vi "WASH communication handler.vi"(7 "task":T2, 8 "error in (no error)":errorcluster, 11 "parameters":variant) -> (0 "error out":errorcluster, 1 "timed out?":bool, 2 "UI data":variant, 3 "UI command":T1)   [LabVIEW 2013]
doc: "Handles communication between controller and console/consoles. It separates controller from console. In subsequent phases of the project only this VI has to be modified to establish communication between controller and the console.\n\n[Covers: SI1]"
uses:
  type defs/WASH communication module tasks.ctl
  type defs/WASH UI to CTRL commands.ctl
  type defs/Wash CTRL to UI message.ctl
  type defs/WASH CTRL to UI commands.ctl
  type defs/WASH UI to CTRL message.ctl
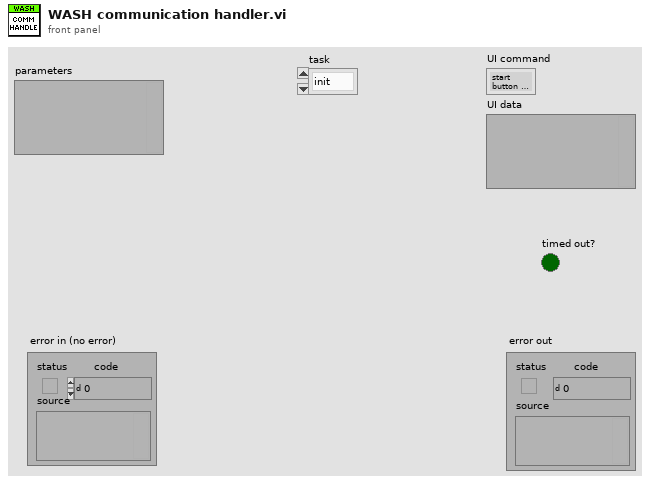
[diagram p1: front panel]
types:
  T1 = typedef "WASH UI to CTRL commands.ctl" = enum16{"start button pushed", "vehicle position changed"}
  T2 = typedef "WASH communication module tasks.ctl" = enum16{"init", "enable controls", "update wash indicators", "update wash entry", "update vehicle out of pos", "update timing", "set step buttons values", "set start button value", "set vehicle position entry", "wait for input", "close"}
  T3 = typedef "Wash CTRL to UI message.ctl" = cluster{"command":T4, "data":variant}
  T4 = typedef "WASH CTRL to UI commands.ctl" = enum16{"enable controls", "set start button value", "update vehicle out of pos", "update wash indicators", "update timing", "set vehicle position entry", "abort"}
  T5 = typedef "WASH UI to CTRL message.ctl" = cluster{"command":T1, "data":variant}
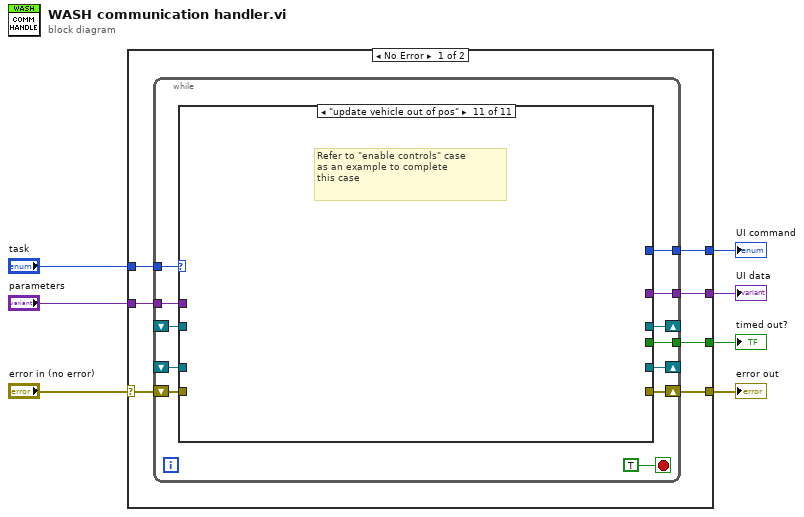
[diagram p0: block diagram]
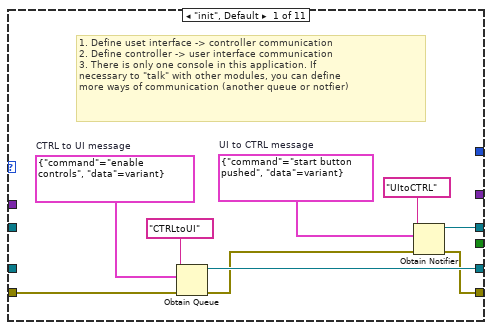
[diagram p2: hidden frame]
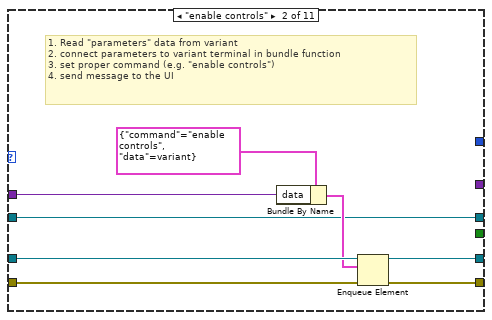
[diagram p3: hidden frame]
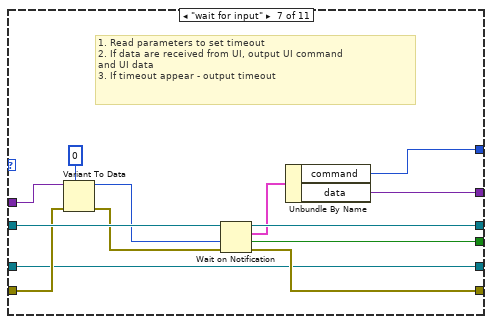
[diagram p8: hidden frame]
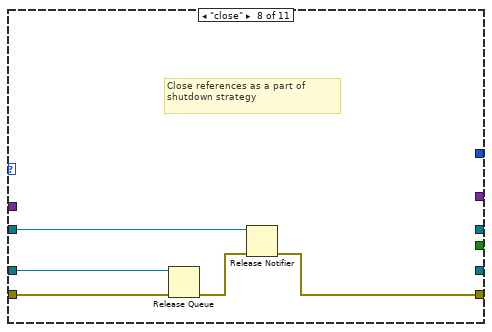
[diagram p9: hidden frame]
diagram:
  n1 = case shown="No Error" "error in (no error)" {
    selector: "error in (no error)" -> [w13 w62]
    tunnel: [w12 w62] -> w6
    tunnel: "task" -> [w14 _]
    tunnel: "parameters" -> [w11 _]
    tunnel: [w10 _] -> w3
    tunnel: [w9 _] -> w2
    tunnel: [w8 _] -> w1
    frame No Error {
      n2 = while {
        tunnel: w14 -> [w25]
        shift-right: [w24] -> _
        shift-left: _ -> [w18]
        shift-right: [w23] -> _
        shift-left: _ -> [w20]
        shift-right: [w21] -> w12
        shift-left: w13 -> [w22]
        tunnel: w11 -> [w19]
        tunnel: [w17] -> w10
        tunnel: [w16] -> w9
        tunnel: [w15] -> w8
        stop <- TRUE stop-if-true
        n3 = case shown="\"update vehicle out of pos\"" w25 {
          tunnel: [w35 w36 _ _ _ _ w55 _ _ _ _] -> w24
          tunnel: [w34 w42 _ _ _ _ w44 _ _ _ _] -> w23
          tunnel: w22 -> [w32 w41 _ _ _ _ w52 w59 _ _ _]
          tunnel: [w31 w40 _ _ _ _ w54 w57 _ _ _] -> w21
          tunnel: w20 -> [_ w43 _ _ _ _ w44 w60 _ _ _]
          tunnel: w19 -> [_ w38 _ _ _ _ w53 _ _ _ _]
          tunnel: w18 -> [_ w36 _ _ _ _ w56 w61 _ _ _]
          tunnel: [_ _ _ _ _ _ w48 _ _ _ _] -> w17
          tunnel: [_ _ _ _ _ _ w46 _ _ _ _] -> w16
          tunnel: [_ _ _ _ _ _ w45 _ _ _ _] -> w15
          frame "init", Default {
            w27 = T5 {"command"=enum."start button pushed", "data"=variant}  # UI to CTRL message
            w28 = T3 {"command"=enum."enable controls", "data"=variant}  # CTRL to UI message
            # "1. Define uset interface -> controller communication\n2. Define controller -> user interface communication\n3. There is only one console in this application. If\nnecessary to \"talk\" with other modules, you can define\nmore ways of communication (another queue or notfier)"
            n4 = Obtain Queue(name (unnamed)="CTRLtoUI", element data type=w28, error in (no error)=w32) -> (queue out=w34:refnum<queue>, error out=w33:errorcluster)  [unwired: 2 in, 1 out]
            n5 = Obtain Notifier(name (unnamed)="UItoCTRL", notification data type=w27, error in (no error)=w33) -> (notifier out=w35:refnum<notifier>, error out=w31:errorcluster)  [unwired: 1 in, 1 out]
          }
          frame "enable controls" {
            # "1. Read \"parameters\" data from variant\n2. connect parameters to variant terminal in bundle function\n3. set proper command (e.g. \"enable controls\")\n4. send message to the UI"
            n6 = Bundle By Name(cluster=T3 {"command"=enum."enable controls", "data"=variant} ("element"), "data"=w38) -> (w37:T3)
            n7 = Enqueue Element(queue=w43, element=w37, error in (no error)=w41) -> (queue out=w42:refnum<queue>, error out=w40:errorcluster)  [unwired: 1 in, 1 out]
          }
          frame "update wash indicators" {
            # "Refer to \"enable controls\" case\nas an example to complete\nthis case"
          }
          frame "update timing" {
            # "Refer to \"enable controls\" case\nas an example to complete\nthis case"
          }
          frame "set start button value" {
            # "Refer to \"enable controls\" case\nas an example to complete\nthis case"
          }
          frame "set vehicle position entry" {
            # "Refer to \"enable controls\" case\nas an example to complete\nthis case"
          }
          frame "wait for input" {
            # "1. Read parameters to set timeout\n2. If data are received from UI, output UI command\nand UI data\n3. If timeout appear - output timeout"
            n8 = Variant To Data(error in=w52, type=0, Variant=w53) -> (data=w49:i32, error out=w51:errorcluster)
            n9 = Wait on Notification(notifier=w56, timeout in ms (-1)=w49, error in (no error)=w51) -> (notifier out=w55:refnum<notifier>, notification=w47:T5, timed out?=w48:bool, error out=w54:errorcluster)  [unwired: 1 in]
            n10 = Unbundle By Name(w47) -> ("command"=w46:T1, "data"=w45:variant)
          }
          frame "close" {
            # "Close references as a part of\nshutdown strategy"
            n11 = Release Queue(queue=w60, error in (no error)=w59) -> (error out=w58:errorcluster)  [unwired: 1 in, 2 out]
            n12 = Release Notifier(notifier=w61, error in (no error)=w58) -> (error out=w57:errorcluster)  [unwired: 1 in, 2 out]
          }
          frame "set step buttons values" {
            # "Refer to \"enable controls\" case\nas an example to complete\nthis case"
          }
          frame "update wash entry" {
            # "Refer to \"enable controls\" case\nas an example to complete\nthis case"
          }
          frame "update vehicle out of pos" {
            # "Refer to \"enable controls\" case\nas an example to complete\nthis case"
          }
        }
      }
    }
    frame Error {
    }
  }
  "error out" <- w6
  "timed out?" <- w3
  "UI command" <- w2
  "UI data" <- w1
